vi "midiOutPlayer.Core.vi"(7 "notifier out":refnum<notifier>, 10 "Track Number":i32, 11 "midiPlayer":refnum<class "midiPlayer.lvclass">) -> ()   [LabVIEW 2020, in "midiPlayer.lvclass"]
uses:
  midiPlayer.lvclass
  midiPlayer.lvclass/midiPlayer.ctl
  shared/midi note number.ctl
  midi-file-event.midi/midi-file-event.midi.lvclass
  C:/code/LabVIEW-MIDI/lv-src/midi-file-event/midi-file-event.lvclass
  midi-file-event.midi/midi-file-event.midi.lvclass/midi-file-event.midi.ctl
  midi-file-event/midi-file-event.lvclass/midi-file-event.ctl
  midi-file-event.midi/MIDI_Messages.get.vi
  midi-file-event/uid.get.vi
  midi-file-event.midi/Data1.get.vi
  9921281b-b4b3-45e8-863f-f332002011e8.vi
  midi-file-event.midi/Data2.get.vi
  midi/midi.lvclass
  midi-ui/midi-ui.lvclass
  midi-file-events/midi-file-events.lvclass
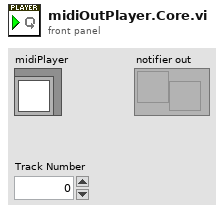
[diagram p1: front panel]
types:
  T1 = typedef "midi note number.ctl" = enum8{"0 - C-1 - 8.18", "1 - C#-1 - 8.66", "2 - D-1 - 9.18", "3 - D#-1 - 9.72", "4 - E-1 - 10.30", "5 - F-1 - 10.91", "6 - F#-1 - 11.56", "7 - G-1 - 12.25", "8 - G#-1 - 12.98", "9 - A-1 - 13.75", "10 - A#-1 - 14.57", "11 - B-1 - 15.43", "12 - C0 - 16.35", "13 - C#0 - 17.32", "14 - D0 - 18.35", "15 - D#0 - 19.45", "16 - E0 - 20.60", "17 - F0 - 21.83", "18 - F#0 - 23.12", "19 - G0 - 24.50", "20 - G#0 - 25.96", "21 - A0 - 27.50", "22 - A#0 - 29.14", "23 - B0 - 30.87", "24 - C1 - 32.70", "25 - C#1 - 34.65", "26 - D1 - 36.71", "27 - D#1 - 38.89", "28 - E1 - 41.20", "29 - F1 - 43.65", "30 - F#1 - 46.25", "31 - G1 - 49.00", "32 - G#1 - 51.91", "33 - A1 - 55.00", "34 - A#1 - 58.27", "35 - B1 - 61.74", "36 - C2 - 65.41", "37 - C#2 - 69.30", "38 - D2 - 73.42", "39 - D#2 - 77.78", "40 - E2 - 82.41", "41 - F2 - 87.31", "42 - F#2 - 92.50", "43 - G2 - 98.00", "44 - G#2 - 103.83", "45 - A2 - 110.00", "46 - A#2 - 116.54", "47 - B2 - 123.47", "48 - C3 - 130.81", "49 - C#3 - 138.59", "50 - D3 - 146.83", "51 - D#3 - 155.56", "52 - E3 - 164.81", "53 - F3 - 174.61", "54 - F#3 - 185.00", "55 - G3 - 196.00", "56 - G#3 - 207.65", "57 - A3 - 220.00", "58 - A#3 - 233.08", "59 - B3 - 246.94", "60 - C4 - 261.63", "61 - C#4 - 277.18", "62 - D4 - 293.66", "63 - D#4 - 311.13", "64 - E4 - 329.63", "65 - F4 - 349.23", "66 - F#4 - 369.99", "67 - G4 - 392.00", "68 - G#4 - 415.30", "69 - A4 - 440.00", "70 - A#4 - 466.16", "71 - B4 - 493.88", "72 - C5 - 523.25", "73 - C#5 - 554.37", "74 - D5 - 587.33", "75 - D#5 - 622.25", "76 - E5 - 659.25", "77 - F5 - 698.46", "78 - F#5 - 739.99", "79 - G5 - 783.99", "80 - G#5 - 830.61", "81 - A5 - 880.00", "82 - A#5 - 932.33", "83 - B5 - 987.77", "84 - C6 - 1046.50", "85 - C#6 - 1108.73", "86 - D6 - 1174.66", "87 - D#6 - 1244.51", "88 - E6 - 1318.51", "89 - F6 - 1396.91", "90 - F#6 - 1479.98", "91 - G6 - 1567.98", "92 - G#6 - 1661.22", "93 - A6 - 1760.00", "94 - A#6 - 1864.66", "95 - B6 - 1975.53", "96 - C7 - 2093.00", "97 - C#7 - 2217.46", "98 - D7 - 2349.32", "99 - D#7 - 2489.02", "100 - E7 - 2637.02", "101 - F7 - 2793.83", "102 - F#7 - 2959.96", "103 - G7 - 3135.96", "104 - G#7 - 3322.44", "105 - A7 - 3520.00", "106 - A#7 - 3729.31", "107 - B7 - 3951.07", "108 - C8 - 4186.01", "109 - C#8 - 4434.92", "110 - D8 - 4698.63", "111 - D#8 - 4978.03", "112 - E8 - 5274.04", "113 - F8 - 5587.65", "114 - F#8 - 5919.91", "115 - G8 - 6271.93", "116 - G#8 - 6644.88", "117 - A8 - 7040.00", "118 - A#8 - 7458.62", "119 - B8 - 7902.13", "120 - C9 - 8372.02", "121 - C#9 - 8869.84", "122 - D9 - 9397.27", "123 - D#9 - 9956.06", "124 - E9 - 10548.08", "125 - F9 - 11175.30", "126 - F#9 - 11839.82", "127 - G9 - 12543.85"}
  T2 = map{T1, refnum<class "midi-file-event.midi.lvclass">}
  T3 = map{dbl, set{refnum<class "midi-file-event.midi.lvclass">}}
  T4 = cluster{"Timestamp":dbl, set{refnum<class "midi-file-event.midi.lvclass">}}[]
  T5 = cluster{"Timestamp":dbl, set{refnum<class "midi-file-event.midi.lvclass">}}
  T6 = set{refnum<class "midi-file-event.midi.lvclass">}
  T7 = typedef "midi-file.lvclass/MIDI Messages.ctl" = enum8{"0(0x00)_UnassignedMidiMessage", "1(0x01)_UnassignedMidiMessage", "2(0x02)_UnassignedMidiMessage", "3(0x03)_UnassignedMidiMessage", "4(0x04)_UnassignedMidiMessage", "5(0x05)_UnassignedMidiMessage", "6(0x06)_UnassignedMidiMessage", "7(0x07)_UnassignedMidiMessage", "8(0x08)_NoteOffEvent", "9(0x09)_NoteOnEvent", "10(0x0A)_PolyphonicKeyPressure", "11(0x0B)_ControlChange", "12(0x0C)_ProgramChange", "13(0x0D)_ChannelPressure", "14(0x0E)_PitchBendChange", "15(0x0F)_SystemExclusive(SysEx)", "16(0x10)_UnassignedMidiMessage", "17(0x11)_UnassignedMidiMessage", "18(0x12)_UnassignedMidiMessage", "19(0x13)_UnassignedMidiMessage", "20(0x14)_UnassignedMidiMessage", "21(0x15)_UnassignedMidiMessage", "22(0x16)_UnassignedMidiMessage", "23(0x17)_UnassignedMidiMessage", "24(0x18)_UnassignedMidiMessage", "25(0x19)_UnassignedMidiMessage", "26(0x1A)_UnassignedMidiMessage", "27(0x1B)_UnassignedMidiMessage", "28(0x1C)_UnassignedMidiMessage", "29(0x1D)_UnassignedMidiMessage", "30(0x1E)_UnassignedMidiMessage", "31(0x1F)_UnassignedMidiMessage", "32(0x20)_UnassignedMidiMessage", "33(0x21)_UnassignedMidiMessage", "34(0x22)_UnassignedMidiMessage", "35(0x23)_UnassignedMidiMessage", "36(0x24)_UnassignedMidiMessage", "37(0x25)_UnassignedMidiMessage", "38(0x26)_UnassignedMidiMessage", "39(0x27)_UnassignedMidiMessage", "40(0x28)_UnassignedMidiMessage", "41(0x29)_UnassignedMidiMessage", "42(0x2A)_UnassignedMidiMessage", "43(0x2B)_UnassignedMidiMessage", "44(0x2C)_UnassignedMidiMessage", "45(0x2D)_UnassignedMidiMessage", "46(0x2E)_UnassignedMidiMessage", "47(0x2F)_UnassignedMidiMessage", "48(0x30)_UnassignedMidiMessage", "49(0x31)_UnassignedMidiMessage", "50(0x32)_UnassignedMidiMessage", "51(0x33)_UnassignedMidiMessage", "52(0x34)_UnassignedMidiMessage", "53(0x35)_UnassignedMidiMessage", "54(0x36)_UnassignedMidiMessage", "55(0x37)_UnassignedMidiMessage", "56(0x38)_UnassignedMidiMessage", "57(0x39)_UnassignedMidiMessage", "58(0x3A)_UnassignedMidiMessage", "59(0x3B)_UnassignedMidiMessage", "60(0x3C)_UnassignedMidiMessage", "61(0x3D)_UnassignedMidiMessage", "62(0x3E)_UnassignedMidiMessage", "63(0x3F)_UnassignedMidiMessage", "64(0x40)_UnassignedMidiMessage", "65(0x41)_UnassignedMidiMessage", "66(0x42)_UnassignedMidiMessage", "67(0x43)_UnassignedMidiMessage", "68(0x44)_UnassignedMidiMessage", "69(0x45)_UnassignedMidiMessage", "70(0x46)_UnassignedMidiMessage", "71(0x47)_UnassignedMidiMessage", "72(0x48)_UnassignedMidiMessage", "73(0x49)_UnassignedMidiMessage", "74(0x4A)_UnassignedMidiMessage", "75(0x4B)_UnassignedMidiMessage", "76(0x4C)_UnassignedMidiMessage", "77(0x4D)_UnassignedMidiMessage", "78(0x4E)_UnassignedMidiMessage", "79(0x4F)_UnassignedMidiMessage", "80(0x50)_UnassignedMidiMessage", "81(0x51)_UnassignedMidiMessage", "82(0x52)_UnassignedMidiMessage", "83(0x53)_UnassignedMidiMessage", "84(0x54)_UnassignedMidiMessage", "85(0x55)_UnassignedMidiMessage", "86(0x56)_UnassignedMidiMessage", "87(0x57)_UnassignedMidiMessage", "88(0x58)_UnassignedMidiMessage", "89(0x59)_UnassignedMidiMessage", "90(0x5A)_UnassignedMidiMessage", "91(0x5B)_UnassignedMidiMessage", "92(0x5C)_UnassignedMidiMessage", "93(0x5D)_UnassignedMidiMessage", "94(0x5E)_UnassignedMidiMessage", "95(0x5F)_UnassignedMidiMessage", "96(0x60)_UnassignedMidiMessage", "97(0x61)_UnassignedMidiMessage", "98(0x62)_UnassignedMidiMessage", "99(0x63)_UnassignedMidiMessage", "100(0x64)_UnassignedMidiMessage", "101(0x65)_UnassignedMidiMessage", "102(0x66)_UnassignedMidiMessage", "103(0x67)_UnassignedMidiMessage", "104(0x68)_UnassignedMidiMessage", "105(0x69)_UnassignedMidiMessage", "106(0x6A)_UnassignedMidiMessage", "107(0x6B)_UnassignedMidiMessage", "108(0x6C)_UnassignedMidiMessage", "109(0x6D)_UnassignedMidiMessage", "110(0x6E)_UnassignedMidiMessage", "111(0x6F)_UnassignedMidiMessage", "112(0x70)_UnassignedMidiMessage", "113(0x71)_UnassignedMidiMessage", "114(0x72)_UnassignedMidiMessage", "115(0x73)_UnassignedMidiMessage", "116(0x74)_UnassignedMidiMessage", "117(0x75)_UnassignedMidiMessage", "118(0x76)_UnassignedMidiMessage", "119(0x77)_UnassignedMidiMessage", "120(0x78)_UnassignedMidiMessage", "121(0x79)_UnassignedMidiMessage", "122(0x7A)_UnassignedMidiMessage", "123(0x7B)_UnassignedMidiMessage", "124(0x7C)_UnassignedMidiMessage", "125(0x7D)_UnassignedMidiMessage", "126(0x7E)_UnassignedMidiMessage", "127(0x7F)_UnassignedMidiMessage"}
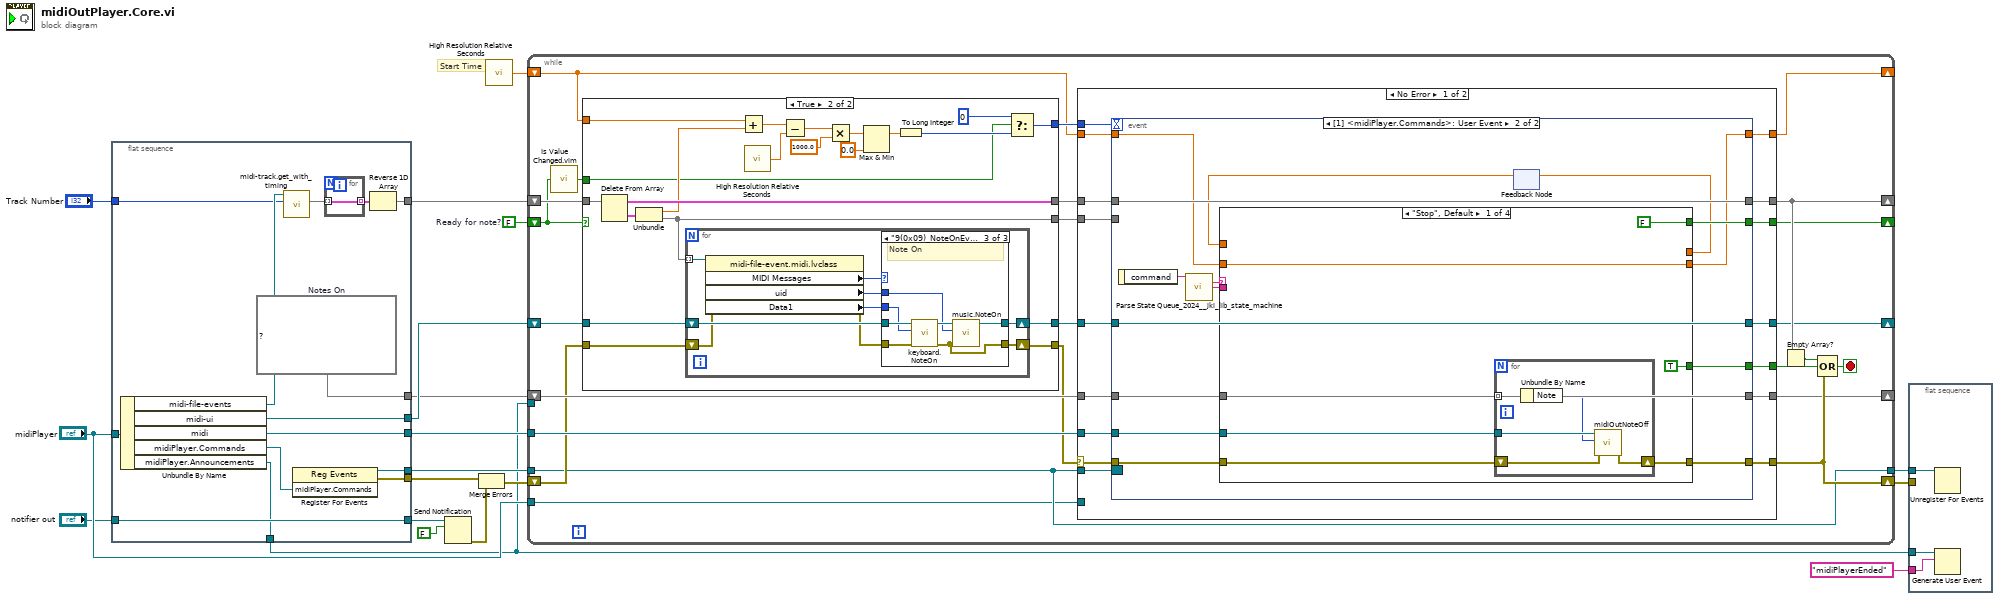
[diagram p0: block diagram]
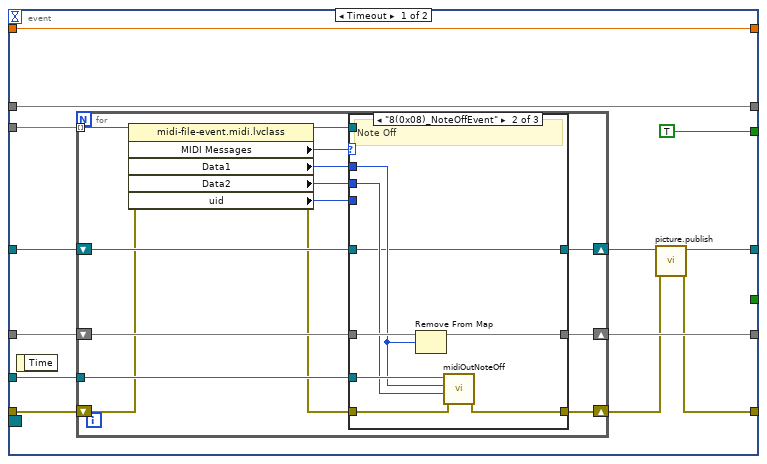
[diagram p2: hidden frame]
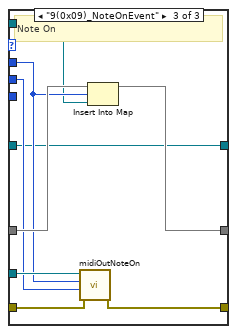
[diagram p4: hidden frame]
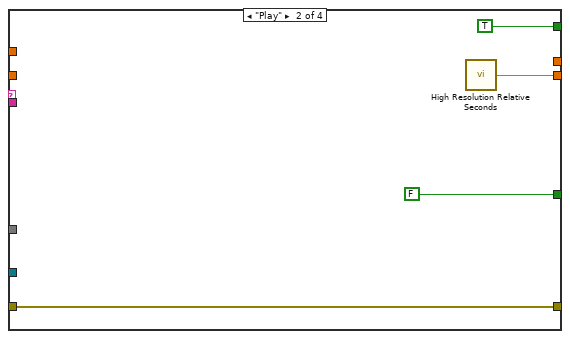
[diagram p5: hidden frame]
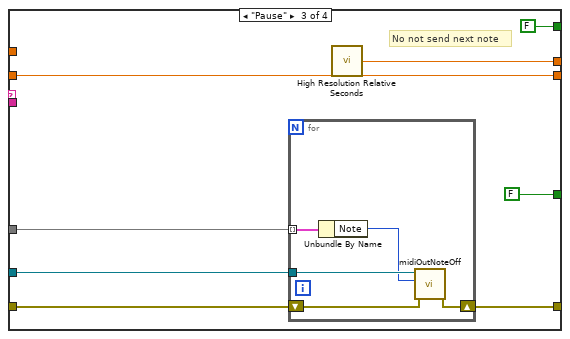
[diagram p6: hidden frame]
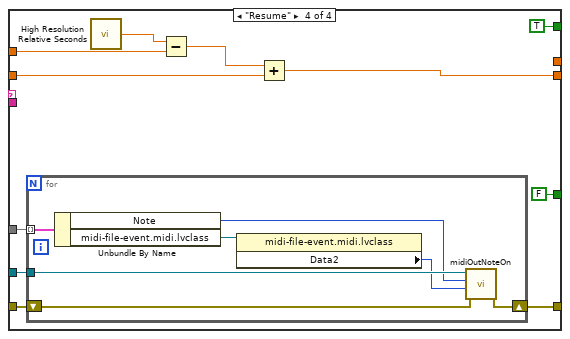
[diagram p7: hidden frame]
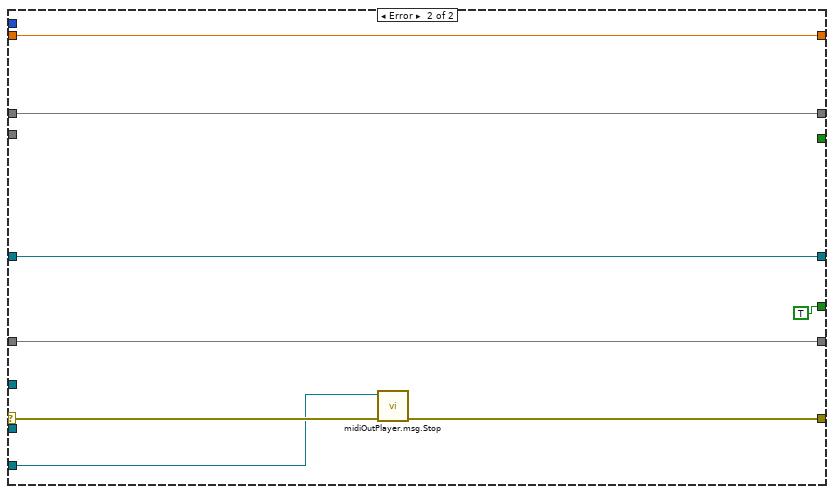
[diagram p8: hidden frame]
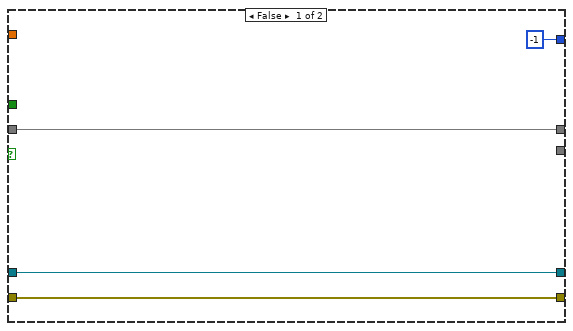
[diagram p9: hidden frame]
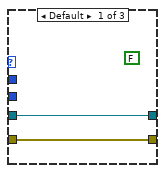
[diagram p10: hidden frame]
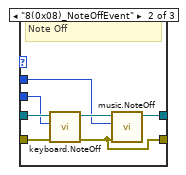
[diagram p11: hidden frame]
diagram:
  w14 = FALSE  # Ready for note?
  # "Start Time"
  n1 = flat-sequence {
    tunnel: [w33] -> w18
    tunnel: [w32] -> w17
    tunnel: [w31] -> w13
    tunnel: [w29] -> w12
    tunnel: [w28] -> w10
    tunnel: "Track Number" -> [w26]
    tunnel: "midiPlayer" -> [w24]
    tunnel: "notifier out" -> [w22]
    tunnel: [w22] -> w4
    tunnel: [w21] -> w3
    tunnel: [w20] -> w2
    frame #0 {
      w21 = T2 {}  # Notes On
      n2 = Unbundle By Name(w24) -> ("midi-file-events"=w27:refnum<class "midi-file-events.lvclass">, "midi-ui"=w29:refnum<class "midi-ui.lvclass">, "midi"=w31:refnum<class "midi.lvclass">, "midiPlayer.Commands"=w30:refnum<user-event>, "midiPlayer.Announcements"=w20:refnum<user-event>)
      n3 = call "midi-track.get_with_timing.vi"("Track Number"=w26, "midi-file-events in"=w27) -> ("Events by time"=w25:T3)  [unwired: 7 in, 2 out]
      n4 = register-events(w30) -> (reference out=w32:refnum<event-registration>, error out=w33:errorcluster)  [unwired: 2 in]
      n5 = for {
        tunnel: w25 -> [w34] mode=indexing
        tunnel: [w34] -> w23 mode=indexing
      }
      n6 = Reverse 1D Array(array=w23) -> (reversed array=w28:T4)
    }
  }
  n7 = Send Notification(notification=FALSE, notifier=w4) -> (error out=w19:errorcluster)  [unwired: 1 in, 1 out]
  n8 = Merge Errors(w18, w19) -> (w16:errorcluster)
  n9 = call <vilib>:"High Resolution Relative Seconds.vi"() -> ("relative seconds"=w11:dbl)
  n10 = while {
    shift-right: [w58] -> _
    shift-left: w10 -> [w50]
    shift-right: [w56] -> w1
    shift-left: w16 -> [w38]
    tunnel: w17 -> [w36]
    tunnel: w13 -> [w54]
    tunnel: w2 -> [_]
    shift-right: [w51] -> _
    shift-left: w3 -> [w52]
    shift-right: [w47] -> _
    shift-left: w14 -> [w40]
    shift-right: [w46] -> _
    shift-left: w12 -> [w45]
    shift-right: [w42] -> _
    shift-left: w11 -> [w41]
    tunnel: [w36] -> w8
    tunnel: "midiPlayer" -> [w35]
    stop <- w55 stop-if-true
    n11 = call "Is Value Changed.vim"("value"=w40) -> ("changed or first call?"=w39:bool)
    n12 = case shown="True" w40 {
      tunnel: w50 -> [w195 w216]
      tunnel: [w195 w215] -> w49
      tunnel: [_ w202] -> w48
      tunnel: w45 -> [w194 w214]
      tunnel: [w194 w213] -> w44
      tunnel: [-1 w200] -> w43
      tunnel: w41 -> [_ w205]
      tunnel: w39 -> [_ w196]
      tunnel: w38 -> [w192 w199]
      tunnel: [w192 w198] -> w37
      frame False {
      }
      frame True {
        n13 = Delete From Array(array=w216) -> (deleted portion=w206:T5, array with subset deleted=w215:T4)  [unwired: 2 in]
        n14 = Unbundle(w206) -> ("Timestamp"=w204:dbl, w202:T6)
        n15 = for {
          tunnel: w202 -> [w223] mode=indexing
          shift-right: [w224] -> w213
          shift-left: w214 -> [w225]
          shift-right: [w219] -> w198
          shift-left: w199 -> [w217]
          n16 = property class="midi-file-event.midi.lvclass"(reference=w223, error in=w217) -> (error out=w218:errorcluster, "MIDI Messages"=w220:T7, "uid"=w221:u64, "Data1"=w222:u8)  [unwired: 1 out]
          n17 = case shown="\"9(0x09)_NoteOnEvent\"" w220 {
            tunnel: w221 -> [_ w231 w240]
            tunnel: w225 -> [w227 w233 w239]
            tunnel: [w227 w232 w238] -> w224
            tunnel: w222 -> [_ w230 w237]
            tunnel: [w226 w228 w235] -> w219
            tunnel: w218 -> [w226 w229 w236]
            frame Default {
              (unwired) FALSE ("status")
            }
            frame "8(0x08)_NoteOffEvent" {
              # "Note Off"
              n18 = call "keyboard.NoteOff.vi"("error in (no error)"=w229, "Note"=w230, "midi-ui in"=w233) -> ("error out"=w228:errorcluster, "midi-ui out"=w234:refnum<class "midi-ui.lvclass">)  [unwired: 7 in]
              n19 = call "music.NoteOff.vi"("error in (no error)"=w228, "uid"=w231, "midi-ui in"=w234) -> ("midi-ui out"=w232:refnum<class "midi-ui.lvclass">)  [unwired: 7 in, 1 out]
            }
            frame "9(0x09)_NoteOnEvent" {
              # "Note On"
              n20 = call "keyboard.NoteOn.vi"("error in (no error)"=w236, "Note"=w237, "midi-ui in"=w239) -> ("error out"=w235:errorcluster, "midi-ui out"=w241:refnum<class "midi-ui.lvclass">)  [unwired: 7 in]
              n21 = call "music.NoteOn.vi"("error in (no error)"=w235, "uid"=w240, "midi-ui in"=w241) -> ("midi-ui out"=w238:refnum<class "midi-ui.lvclass">)  [unwired: 7 in, 1 out]
            }
          }
        }
        n22 = Add(x=w205, y=w204) -> (x+y=w203:dbl)
        n23 = call <vilib>:"High Resolution Relative Seconds.vi"() -> ("relative seconds"=w212:dbl)
        n24 = Subtract(x=w203, y=w212) -> (x-y=w211:dbl)
        n25 = Multiply(x=w211, y=1000.0) -> (x*y=w209:dbl)
        n26 = Max & Min(x=w209, y=0.0) -> (max(x,y)=w207:dbl)  [unwired: 1 out]
        n27 = To Long Integer(number=w207) -> (32bit integer=w201:i32)
        n28 = Select(t=0, s=w196, f=w201) -> (s? t:f=w200:i32)
      }
    }
    n29 = case shown="No Error" w37 {
      selector: w37 -> [w59 w186]
      tunnel: [w74 w188] -> w58
      tunnel: [w73 w185] -> w56
      tunnel: w36 -> [w72 _]
      tunnel: w54 -> [w71 _]
      tunnel: [w70 TRUE] -> w53
      tunnel: w52 -> [w69 w190]
      tunnel: [w68 w190] -> w51
      tunnel: w49 -> [w67 w188]
      tunnel: w48 -> [w66 _]
      tunnel: [w65 _] -> w47
      tunnel: [w64 w189] -> w46
      tunnel: w44 -> [w63 w189]
      tunnel: w43 -> [w62 _]
      tunnel: [w61 w187] -> w42
      tunnel: w41 -> [w60 w187]
      tunnel: w35 -> [_ w184]
      frame No Error {
        n30 = event shown="[1] <midiPlayer.Commands>: User Event" {
          selector: w72 -> [_ _]
          dyn-events: _ -> [_ _]
          timeout: w62 -> [_ _]
          tunnel: w71 -> [w87 w129]
          tunnel: w59 -> [w86 w134]
          tunnel: w67 -> [w76 w136]
          tunnel: [w76 w136] -> w74
          tunnel: [w77 w135] -> w73
          tunnel: [_ w133] -> w70
          tunnel: w69 -> [w85 w122]
          tunnel: [w84 w122] -> w68
          tunnel: w66 -> [w75 _]
          tunnel: [TRUE w128] -> w65
          tunnel: w63 -> [w82 w127]
          tunnel: [w79 w127] -> w64
          tunnel: [w81 w126] -> w61
          tunnel: w60 -> [w81 w125]
          event Timeout {
            n31 = event-data() -> ()  [unwired: 1 in, 1 out]
            n32 = for {
              tunnel: w87 -> [w101]
              shift-right: [w92] -> w78
              shift-left: w86 -> [w89]
              shift-right: [w93] -> w80
              shift-left: w82 -> [w98]
              shift-right: [w99] -> w84
              shift-left: w85 -> [w100]
              tunnel: w75 -> [w91] mode=indexing
              n33 = property class="midi-file-event.midi.lvclass"(reference=w91, error in=w89) -> (reference out=w90:refnum<class "midi-file-event.midi.lvclass">, error out=w88:errorcluster, "MIDI Messages"=w94:T7, "Data1"=w97:u8, "Data2"=w96:u8, "uid"=w95:u64)
              n34 = case shown="\"8(0x08)_NoteOffEvent\"" w94 {
                tunnel: w101 -> [_ w112 w121]
                tunnel: w97 -> [_ w107 w116]
                tunnel: w96 -> [_ w106 w115]
                tunnel: w88 -> [w104 w111 w117]
                tunnel: [w104 w108 w120] -> w92
                tunnel: w100 -> [w103 w110 w119]
                tunnel: [w103 w109 w118] -> w99
                tunnel: w95 -> [_ _ _]
                tunnel: w98 -> [w102 w105 w114]
                tunnel: [w102 w105 w114] -> w93
                tunnel: w90 -> [_ _ w113]
                frame Default {
                }
                frame "8(0x08)_NoteOffEvent" {
                  # "Note Off"
                  n35 = Remove From Map(10:w107, 11:w110) -> (3:w109:T2)  [unwired: 2 out]
                  n36 = call "midiOutNoteOff.vi"("error in"=w111, "Velocity (0-127)"=w106, "Note"=w107, "midi in"=w112) -> ("error out"=w108:errorcluster)  [unwired: 6 in, 1 out]
                }
                frame "9(0x09)_NoteOnEvent" {
                  # "Note On"
                  n37 = call "midiOutNoteOn.vi"("error in"=w117, "Velocity (0-127)"=w115, "Note"=w116, "midi in"=w121) -> ("error out"=w120:errorcluster)  [unwired: 6 in, 1 out]
                  n38 = Insert Into Map(map in=w119, key=w116, value=w113) -> (map out=w118:T2)  [unwired: 2 out]
                }
              }
            }
            n39 = call "picture.publish.vi"("error in"=w78, "midi-ui in"=w80) -> ("error out"=w77:errorcluster, "midi-ui out"=w79:refnum<class "midi-ui.lvclass">)  [unwired: 8 in]
          }
          event User Event {
            n40 = event-data() -> ("command"=w132:string)  [unwired: 1 in]
            n41 = call <vilib>:"Parse State Queue_2024__jki_lib_state_machine.vi"("State Queue"=w132) -> ("Current State"=w131:string, "Arguments"=w130:string)  [unwired: 12 in, 1 out]
            n42 = feedback #1() -> (w123:dbl)  [unwired: 1 in]
            n43 = case shown="\"Stop\", Default" w131 {
              tunnel: [w140 w151 w156 w172] -> w135
              tunnel: w134 -> [w141 w151 w157 w173]
              tunnel: [TRUE FALSE FALSE FALSE] -> w133
              tunnel: w130 -> [_ _ _ _]
              tunnel: w122 -> [w142 _ w158 w174]
              tunnel: w129 -> [w139 _ w159 w175]
              tunnel: [FALSE TRUE FALSE TRUE] -> w128
              tunnel: [w137 w149 w154 w166] -> w126
              tunnel: w125 -> [w137 _ w154 w167]
              tunnel: [_ _ w153 _] -> w124
              tunnel: w123 -> [_ _ _ w169]
              frame "Stop", Default {
                n44 = for {
                  tunnel: w139 -> [w148]
                  tunnel: w142 -> [w147] mode=indexing
                  shift-right: [w144] -> w140
                  shift-left: w141 -> [w145]
                  n45 = Unbundle By Name(w147) -> ("Note"=w146:T1)
                  n46 = call "midiOutNoteOff.vi"("error in"=w145, "Note"=w146, "midi in"=w148) -> ("error out"=w144:errorcluster)  [unwired: 7 in, 1 out]
                }
              }
              frame "Play" {
                n47 = call <vilib>:"High Resolution Relative Seconds.vi"() -> ("relative seconds"=w149:dbl)
              }
              frame "Pause" {
                # "No not send next note"
                n48 = for {
                  tunnel: w159 -> [w165]
                  tunnel: w158 -> [w164] mode=indexing
                  shift-right: [w161] -> w156
                  shift-left: w157 -> [w162]
                  n49 = Unbundle By Name(w164) -> ("Note"=w163:T1)
                  n50 = call "midiOutNoteOff.vi"("error in"=w162, "Note"=w163, "midi in"=w165) -> ("error out"=w161:errorcluster)  [unwired: 7 in, 1 out]
                }
                n51 = call <vilib>:"High Resolution Relative Seconds.vi"() -> ("relative seconds"=w153:dbl)
              }
              frame "Resume" {
                n52 = for {
                  tunnel: w175 -> [w182]
                  tunnel: w174 -> [w183] mode=indexing
                  shift-right: [w180] -> w172
                  shift-left: w173 -> [w181]
                  n53 = Unbundle By Name(w183) -> ("Note"=w177:T1, "midi-file-event.midi.lvclass"=w179:refnum<class "midi-file-event.midi.lvclass">)
                  n54 = property class="midi-file-event.midi.lvclass"(reference=w179) -> ("Data2"=w178:u8)  [unwired: 1 in, 2 out]
                  n55 = call "midiOutNoteOn.vi"("error in"=w181, "Velocity (0-127)"=w178, "Note"=w177, "midi in"=w182) -> ("error out"=w180:errorcluster)  [unwired: 6 in, 1 out]
                }
                n56 = call <vilib>:"High Resolution Relative Seconds.vi"() -> ("relative seconds"=w170:dbl)
                n57 = Subtract(x=w170, y=w169) -> (x-y=w168:dbl)
                n58 = Add(x=w168, y=w167) -> (x+y=w166:dbl)
              }
            }
            n59 = feedback-in #1(w124) -> ()
          }
        }
      }
      frame Error {
        n60 = call "midiOutPlayer.msg.Stop.vi"("error in (no error)"=w186, "midiPlayer in"=w184) -> ("error out"=w185:errorcluster)  [unwired: 8 in, 1 out]
      }
    }
    n61 = Empty Array?(array=w58) -> (empty?=w57:bool)
    n62 = Compound Arithmetic op=OR(w57, w53, w56) -> (w55:bool)
  }
  n63 = flat-sequence {
    tunnel: w2 -> [w244]
    tunnel: "midiPlayerEnded" ("event data") -> [w243]
    tunnel: w8 -> [w242]
    tunnel: w1 -> [_]
    frame #0 {
      n64 = Unregister For Events(event registration refnum=w242) -> ()  [unwired: 1 in, 1 out]
      n65 = Generate User Event(user event=w244, event data cluster=w243) -> ()  [unwired: 2 in, 2 out]
    }
  }
